vi "CommandCycle_FAST.vi"(8 "Gripper Value R":dbl=324.0, 9 "Gripper Value L":dbl=584.0, 10 "Elevator Value":dbl=3.1212669283918144, 11 "Teir Selection":T2) -> (3 "appended array":cluster{"States":T1, "Close":dbl[]}[](array[cluster])=[{"States"=enum."Set Elevator SP", "Close"=[0.49000000000000005, -1.0]}, {"States"=enum."Wait For Elevator Fast", "Close"=[2.17, -1.0]}, {"States"=enum."Set Gripper SP", "Close"=[452.0, 428.0]}, {"States"=enum."Wait For Elevator", "Close"=[0.49000000000000005, -1.0]}, {"States"=enum."Set Gripper SP", "Close"=[592.0, 308.0]}, {"States"=enum."Wait ms", "Close"=[400.0]}, {"States"=enum."Set Elevator SP", "Close"=[3.19]}])   [LabVIEW 2014, in "Elevator System.lvlib"]
uses:
  Elevator System.lvlib
  Typedef/ControllerStates.ctl
  Typedef/TeirNumber.ctl
  Public/StupidGlobal.vi
panel:
  in  "Fudge Factor":dbl=0.08
  in  "Timer ms":dbl=400.0 format="%#_13g"
  in  "Fudge Factor":dbl
  out "appended array":cluster{"States":T1, "Numeric":dbl}[](array[cluster])
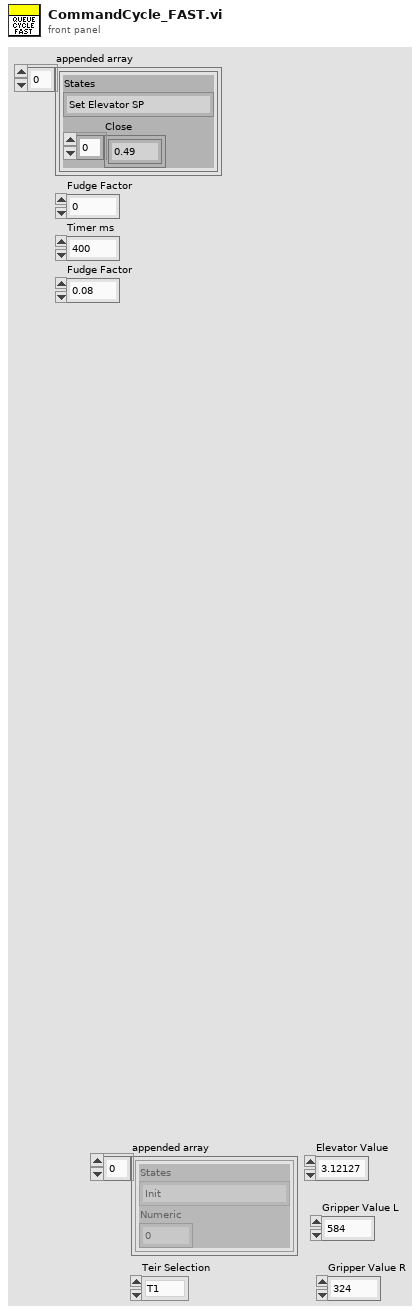
[diagram p1: front panel]
types:
  T1 = typedef "Elevator System.lvlib/ControllerStates.ctl" = enum16{"Init", "Set Elevator SP", "Set Gripper SP", "Wait For Elevator", "Wait For Gripper", "Wait For Elevator Fast", "Wait For Gripper Fast", "Wait ms", "Disabled"}
  T2 = typedef "Elevator System.lvlib/TeirNumber.ctl" = enum16{"T1", "T2", "T3", "T4", "T5", "T6"}
  T3 = typedef "Elevator System.lvlib/GripperNotifierType.ctl" = cluster{"SP Left":dbl, "SP Right":dbl}
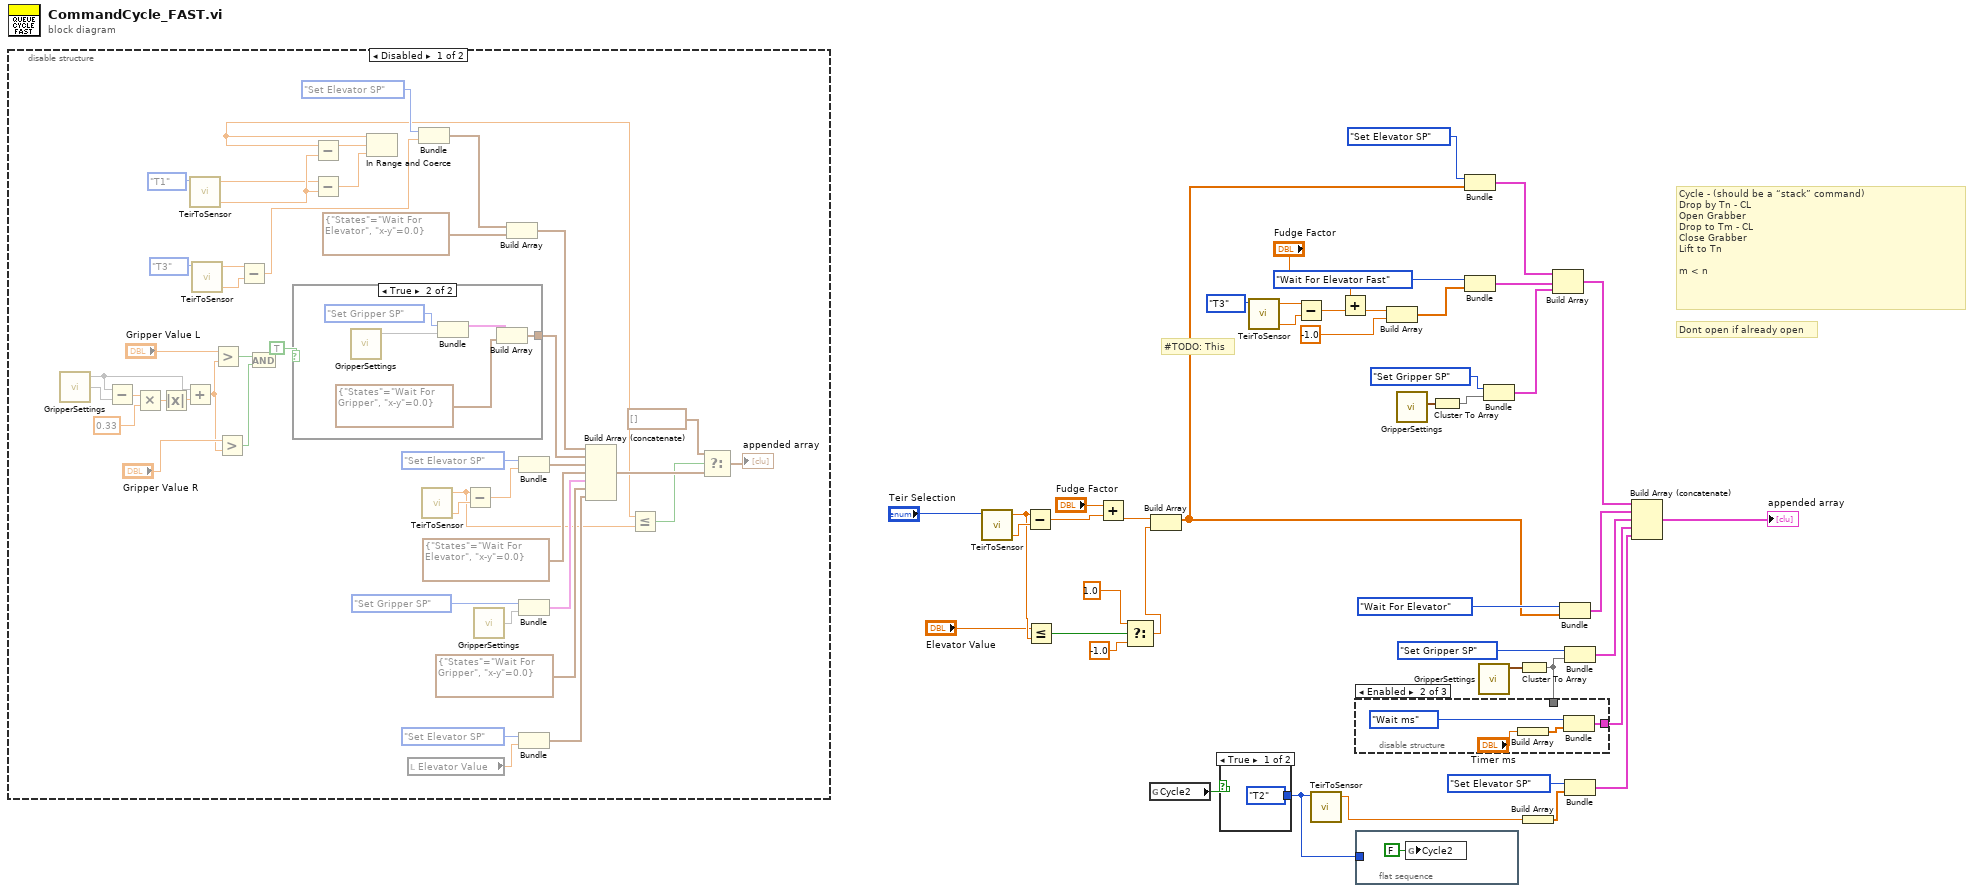
[diagram p0: block diagram]
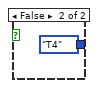
[diagram p2: hidden frame]
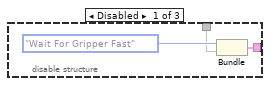
[diagram p3: hidden frame]
diagram:
  # "#TODO: This"
  # "Dont open if already open"
  # "Cycle - (should be a “stack” command)\nDrop by Tn - CL\nOpen Grabber\nDrop to Tm - CL\nClose Grabber\nLift to Tn\n\nm < n"
  n1 = disable-structure shown="Disabled" {
    frame Disabled {
      n2 = call "GripperSettings.vi"() -> (2:w74, 3:w69)  [unwired: 3 in]
      n3 = Subtract(x=w74, y=w69) -> (x-y=w70:dbl)
      n4 = Multiply(x=w70, y=0.33) -> (x*y=w72:dbl)
      n5 = Absolute Value(x=w72) -> (abs(x)=w73:dbl)
      n6 = Add(x=w74, y=w73) -> (x+y=w56:dbl)
      n7 = call "TeirToSensor.vi"("Enum"=TeirNumber."T1") -> ("T1"=w75:dbl, "CL"=w76:dbl)  [unwired: 3 in, 3 out]
      n8 = call "TeirToSensor.vi"("Enum"=TeirNumber."T3") -> ("T1"=w46:dbl, "CL"=w45:dbl)  [unwired: 3 in, 3 out]
      n9 = Greater?(x="Gripper Value L", y=w56) -> (0:w61:bool)
      n10 = Greater?(x="Gripper Value R", y=w56) -> (0:w55:bool)
      n11 = Subtract(x=w46, y=w45) -> (x-y=w44:dbl)
      n12 = And(x=w61, y=w55) -> ()  [unwired: 1 out]
      n13 = case shown="True" TRUE {
        tunnel: [_ w91] -> w62
        frame False {
        }
        frame True {
          n14 = call "GripperSettings.vi"() -> (2:w92)  [unwired: 4 in]
          n15 = Bundle("States"=ControllerStates."Set Gripper SP", w92) -> (w90:cluster{"States":T1, void})  [unwired: 1 in]
          n16 = Build Array(w90, cluster{"States":T1, "x-y":dbl} {"States"=enum."Wait For Gripper", "x-y"=0.0}) -> (w91:cluster{"States":T1, "x-y":dbl}[])
        }
      }
      n17 = Subtract(x=w75, y=w76) -> (x-y=w65:dbl)
      n18 = local read "Elevator Value"() -> (w58:dbl)
      n19 = Bundle("States"=ControllerStates."Set Elevator SP", w44) -> (w64:cluster{"States":T1, dbl})  [unwired: 1 in]
      n20 = call "TeirToSensor.vi"() -> ("Enum"=w59:T2, "T1"=w49:dbl, "CL"=w86:dbl)  [unwired: 3 in, 3 out]
      n21 = Subtract(x=w49, y=w86) -> (x-y=w85:dbl)
      n22 = call "GripperSettings.vi"() -> (3:w80)  [unwired: 4 in]
      n23 = Build Array(w64, cluster{"States":T1, "x-y":dbl} {"States"=enum."Wait For Elevator", "x-y"=0.0}) -> (w77:cluster{"States":T1, "x-y":dbl}[])
      n24 = Bundle("States"=ControllerStates."Set Elevator SP", w85) -> (w83:cluster{"States":T1, dbl})  [unwired: 1 in]
      n25 = Bundle("States"=ControllerStates."Set Gripper SP", w80) -> (w81:cluster{"States":T1, void})  [unwired: 1 in]
      n26 = Bundle("States"=ControllerStates."Set Elevator SP", "Elevator Value"=w58) -> (w88:cluster{"States":T1, "Elevator Value":dbl})  [unwired: 1 in]
      n27 = Build Array (concatenate)(w77, w62, w83, cluster{"States":T1, "x-y":dbl} {"States"=enum."Wait For Elevator", "x-y"=0.0}, w81, cluster{"States":T1, "x-y":dbl} {"States"=enum."Wait For Gripper", "x-y"=0.0}, w88) -> (w53:cluster{"States":T1, "Elevator Value":dbl}[])
      n28 = Subtract(x=w50, y=w76) -> (x-y=w66:dbl)
      n29 = In Range and Coerce(x=w66, lower limit=w65) -> (upper limit=w50:dbl)  [unwired: 2 out]
      n30 = Less Or Equal?(x=w50, y=w49) -> (x <= y?=w52:bool)
      n31 = Select(t=cluster{"States":T1, "Elevator Value":dbl}[] [], s=w52, f=w53) -> (s? t:f=→"appended array":cluster{"States":T1, "Elevator Value":dbl}[])
    }
    frame Enabled {
    }
  }
  n32 = call "TeirToSensor.vi"("Enum"="Teir Selection") -> ("T1"=w23:dbl, "CL"=w41:dbl)  [unwired: 3 in, 3 out]
  n33 = Subtract(x=w23, y=w41) -> (x-y=w40:dbl)
  n34 = Less Or Equal?(x="Elevator Value", y=w23) -> (x <= y?=w10:bool)
  n35 = Add(x="Fudge Factor", y=w40) -> (x+y=w6:dbl)
  n36 = Select(t=1.0 ("element"), s=w10, f=-1.0 ("element")) -> (s? t:f=w7:dbl)
  n37 = global read "StupidGlobal.vi" "Cycle2"() -> (w4:bool)
  n38 = Build Array(w6, w7) -> (w13:dbl[])
  n39 = case shown="True" w4 {
    tunnel: [TeirNumber."T2" ("Enum") TeirNumber."T4" ("Enum")] -> w3
    frame True {
    }
    frame False {
    }
  }
  n40 = call "TeirToSensor.vi"("Enum"=TeirNumber."T3") -> ("T1"=w28:dbl, "CL"=w27:dbl)  [unwired: 3 in, 3 out]
  n41 = Subtract(x=w28, y=w27) -> (x-y=w26:dbl)
  n42 = call "TeirToSensor.vi"("Enum"=w3) -> ("T1"=w11:dbl)  [unwired: 3 in, 4 out]
  n43 = Add(x="Fudge Factor", y=w26) -> (x+y=w2:dbl)
  n44 = flat-sequence {
    tunnel: w3 -> [_]
    frame #0 {
      n45 = global write "StupidGlobal.vi" "Cycle2"(FALSE ("Cycle2")) -> ()
    }
  }
  n46 = Build Array(w2, -1.0 ("element")) -> (w19:dbl[])
  n47 = call "GripperSettings.vi"() -> ("Open"=w30:T3)  [unwired: 5 in, 4 out]
  n48 = Cluster To Array(cluster=w30) -> (array=w18:dbl[])
  n49 = Bundle("States"=ControllerStates."Set Elevator SP", w13) -> (w33:cluster{"States":T1, dbl[]})  [unwired: 1 in]
  n50 = Bundle("States"=ControllerStates."Wait For Elevator Fast", w19) -> (w20:cluster{"States":T1, dbl[]})  [unwired: 1 in]
  n51 = call "GripperSettings.vi"() -> ("Close"=w36:T3)  [unwired: 5 in, 4 out]
  n52 = Bundle("States"=ControllerStates."Set Gripper SP", "Open"=w18) -> (w32:cluster{"States":T1, "Open":dbl[]})  [unwired: 1 in]
  n53 = Cluster To Array(cluster=w36) -> (array=w14:dbl[])
  n54 = disable-structure shown="Enabled" {
    disable-tunnel: [w98 w102 _] -> w15
    disable-tunnel: w14 -> [w97 _ _]
    frame Disabled {
      n55 = Bundle("States"=ControllerStates."Wait For Gripper Fast", "Close"=w97) -> (w98:cluster{"States":T1, "Close":dbl[]})  [unwired: 1 in]
    }
    frame Enabled {
      n56 = Build Array("Timer ms") -> (w101:dbl[])
      n57 = Bundle("States"=ControllerStates."Wait ms", w101) -> (w102:cluster{"States":T1, dbl[]})  [unwired: 1 in]
    }
    frame Disabled {
    }
  }
  n58 = Build Array(w11) -> (w35:dbl[])
  n59 = Build Array(w33, w20, w32) -> (w37:cluster{"States":T1, "Open":dbl[]}[])
  n60 = Bundle("States"=ControllerStates."Wait For Elevator", w13) -> (w16:cluster{"States":T1, dbl[]})  [unwired: 1 in]
  n61 = Bundle("States"=ControllerStates."Set Gripper SP", "Close"=w14) -> (w38:cluster{"States":T1, "Close":dbl[]})  [unwired: 1 in]
  n62 = Bundle("States"=ControllerStates."Set Elevator SP", w35) -> (w43:cluster{"States":T1, dbl[]})  [unwired: 1 in]
  n63 = Build Array (concatenate)(w37, w16, w38, w15, w43) -> (→"appended array":cluster{"States":T1, "Close":dbl[]}[])
